vi "Is Published.vi"(8 "error in (no error)":errorcluster, 11 "Group in":refnum<class "Group Config.lvclass">) -> (0 "error out":errorcluster, 2 "Is Published":bool, 3 "Group out":refnum<class "Group Config.lvclass">)   [LabVIEW 2020, in "VolatusConfig.lvlib" / "Group Config.lvclass"]
uses:
  Group Config.lvclass
  Group Config.lvclass/Group Config.ctl
  VolatusConfigElement/VolatusConfigElement.lvclass
  C:/dev/lv20CE/relink/lv-volatus/VolatusConfig/VolatusConfigElement/VolatusConfigElement.lvclass
  C:/dev/lv20CE/relink/lv-volatus/VolatusConfig/Group/Group Config.lvclass
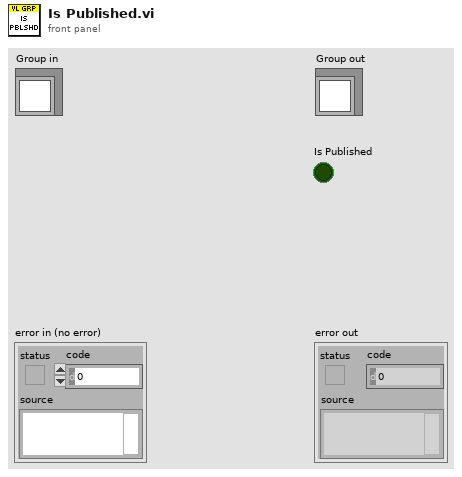
[diagram p1: front panel]
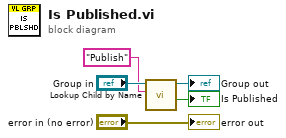
[diagram p0: block diagram]
diagram:
  n1 = call "Lookup Child by Name.vi"("Child Name"="Publish", "VolatusConfigElement in"="Group in") -> ("Found"=→"Is Published":bool, "VolatusConfigElement out"=→"Group out":refnum<class "Group Config.lvclass">)  [unwired: 6 in, 2 out]
  "error out" <- "error in (no error)"
